vi "File or directory exists.vi"(8 "error in (no error)":errorcluster, 10 "Path":string, 11 "File Transfer Behavior in":refnum<class "File Transfer Behavior.lvclass">) -> (0 "error out":errorcluster, 1 "Exists?":bool, 2 "Path out (dup)":string, 3 "File Transfer Behavior out":refnum<class "File Transfer Behavior.lvclass">, 4 "Type":T1)   [LabVIEW 2015, in "RT Management.lvlib" / "File Transfer Behavior.lvclass"]
doc: "Checks to see if the file or directory at \"Path\" exists or not.\n\nThe recommended file path format for \"Path\" is \"/directory1/directory2\" or \"/directory/file.extension\". However, the VI will accept other formats and transform the path appropriately in most cases. Use the \"Strip path.vi\" and \"Build path.vi\" VIs to help with handling remote path strings."
uses:
  File Transfer Behavior.lvclass
  Type.ctl
  RT Management.lvlib
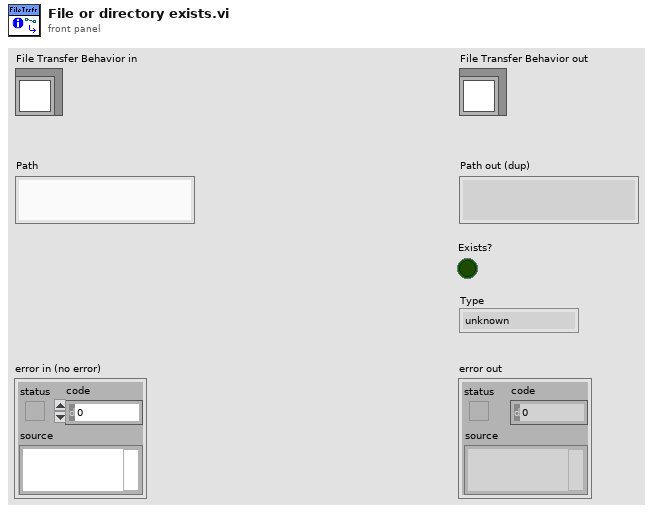
[diagram p1: front panel]
types:
  T1 = typedef "RT Management.lvlib/File Transfer Behavior.lvclass/Type.ctl" = enum16{"unknown", "file", "directory"}
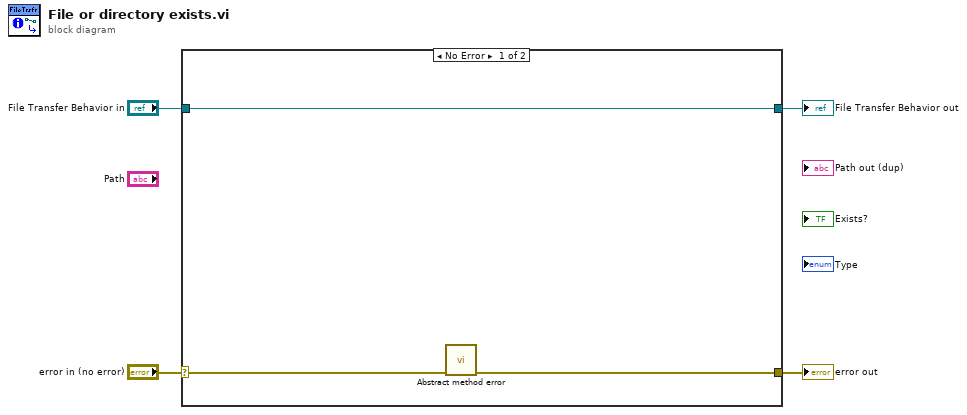
[diagram p0: block diagram]
diagram:
  n1 = case shown="No Error" "error in (no error)" {
    selector: "error in (no error)" -> [w6 w9]
    tunnel: [w5 w9] -> w3
    tunnel: [w7 w8] -> w1
    tunnel: "File Transfer Behavior in" -> [w7 w8]
    frame No Error {
      n2 = call "Abstract method error.vi"("error in (no error)"=w6) -> ("error out"=w5:errorcluster)  [unwired: 10 in]
    }
    frame Error {
    }
  }
  "error out" <- w3
  "File Transfer Behavior out" <- w1
